vi "Debugl Loop Dialog.vi"(1 "Debug W1":u16, 2 "Debug W2":u16, 11 "error in (no error)":errorcluster) -> ()   [LabVIEW 2011]
uses:
  emi Lib/System 01/0 - General/App/Loop control/Private/_emi Loop status.ctl
  PCP interface/PCP Command Return.ctl
  PCP interface/PCP Commands.ctl
  emi Lib/System 01/0 - General/S&E reporting/Private/_emi_ S&E Message.ctl
  emi Lib/System 01/0 - General/S&E reporting/Private/_emi_ S&E Message type.ctl
  emi cndiates/E&S/Monitor/Actino S&E monitor.ctl
  PCP interface/PCP return data types/RDd return.ctl
  PCP interface/PCP return data types/RA return Analog I.ctl
  PCP interface/PCP return data types/RP return digital IO.ctl
  LEINmaster/Defenitions/LEIN CMD List.ctl
  Loop ID.ctl
  Measurments Handling/Action Analog Handler.ctl
  emi cndiates/E&S/String outpyt type.ctl
  PCP interface/PCP Command definer.ctl
  LEINmaster/Defenitions/LEIN Structure variations.ctl
  Options/Action GFV Settings.ctl
  Options/Options PageID.ctl
  emi Lib/System 01/0 - General/App/Loop control 2/Private/_emi_SMLoop Get State Single.vi
  emi Lib/System 01/0 - General/App/Loop control 2/Private/_emi_SMLoop Control Single.vi
  emi Lib/System 01/0 - General/App/Loop control 2/Private/_emi_ SMLoop start condition.vi
  emi Lib/System 01/0 - General/App/Loop control 2/Private/_emi_ SMLoop Error Check.vi
  emi Lib/Basic/0 - General/Error/emi_Is Error.vi
  emi Lib/System 01/0 - General/App/Loop control 2/Private/_emi_SMLoop Register new.vi
  emi Lib/Basic/0 - General/Data Types/emi_Enum Info.vi
  emi Lib/System 01/0 - General/S&E reporting/emi_Send S&E Error message.vi
  emi Lib/Basic/0 - General/Error/emi_ Is Error state.vi
  emi Lib/System 01/0 - General/emi_Read System ID.vi
  emi Lib/System 01/0 - General/App/Loop control/Private/_emi_GFV Loop Running.vi
  emi Lib/System 01/0 - General/App/Loop control/Private/_emi_GFV Loop Enable.vi
  emi Lib/System 01/0 - General/App/Loop control/Private/_emi_GFV Loop Linking.vi
  emi Lib/System 01/0 - General/App/Loop control 2/Private/_emi_ SMLoop Restart.vi
  emi Lib/System 01/0 - General/App/Loop control/Private/_emi_GFV stop a loop so it can reset.vi
  emi Lib/System 01/0 - General/App/Loop control 2/Private/_emi_ SMLoop Restart Counter.vi
  emi Lib/System 01/0 - General/App/Private/_emi_GFV App Close.vi
  emi Lib/System 01/0 - General/Private/_emi_GFV System ID.vi
  emi Lib/System 01/0 - General/S&E reporting/Private/_emi_S&E Q Generator.vi
  emi Lib/System 01/0 - General/Debug/Private/_emi_GFV Debug Disp.vi
  <vilib>/Utility/VariantDataType/GetNumericInfo.vi
  emi Lib/Basic/0 - General/Time/Private/emi_Time offset holder.vi
  emi Lib/System 01/0 - General/Debug/Private/_emi_GFV Debug Aditional.vi
  emi Lib/System 01/0 - General/Debug/Private/_emi_GFV Debug Log.vi
panel:
  in  "Tab Control":T1(tab)
  in  "Send to PCP":bool
  in  "d":dbl
  in  "n":i32
  out "PCP Ans Q. Element":i32
  out "PCP CMD Q. Element":i32
  out "latest notification":T2
  in  "Action":T3
  out "PCP Data out":T4
  out "ms since last data":u32
  in  "Empty":bool
  out "received/timedout 2":timestamp
  out "Valid reply":bool
  in  "Retry on err":bool=TRUE
  out "Receive ACK":bool
  out "motor timeout":bool
  out "Received command":T7
  out "motor returned":bool
  out "received/timedout":timestamp
  out "Received":u8[](array[numeric]) format="%02x"
  out "Time Stamp":timestamp
  out "Sent":u8[](array[numeric]) format="%02x"
  in  "To send (post A/S/T ID)":u8[](array[numeric]) format="%02x"
  in  "ACTI/STAT/TASK ID":u8 format="%02x"
  in  "CMD":T7
  in  "Sub node address":u8 format="%.0x"
  in  "Main controll address":u8=42
  in  "Send to sub node":bool
  in  "Send custom message":bool
  out "Til Tool cmd Q":i32
  out "Tool reply Q":i32
  in  "Sub Timeout (ms)":u16=200
  in  "priority":bool=TRUE
  out "S&E":T8[](array[typedef])
  in  "Action(GET)":T10=enum."Get All"
  in  "Type":T9
  out "size(s)":i32
  out "Alarma":string[](array[string])
  out "Errors":string[](array[string])
  in  "Test error Loop 2":errorcluster
  in  "Trigger 1":bool
  in  "Test error Loop 1":errorcluster
  out "error out":errorcluster
  out "Loops":T11[](array[typedef])
  # "Main controller Stroker: 42\nSolenoid: 16 \nPressure 1: 48 \nPressure 2: 49"
  # "X"
  # "X+1"
  # "X+2"
  # "X+3"
  # "X+4"
  # "X+5"
  # "X+6"
  # "X+7"
  # "X"
  # "X+1"
  # "X+2"
  # "X+3"
  # "X+4"
  # "X+5"
  # "X+6"
  # "X+7"
  # "X+8"
  # "X+9"
  # "X"
  # "X+1"
  # "X+2"
  # "X+3"
  # "X+4"
  # "X+5"
  # "X+6"
  # "X+7"
  # "X+8"
  # "X+9"
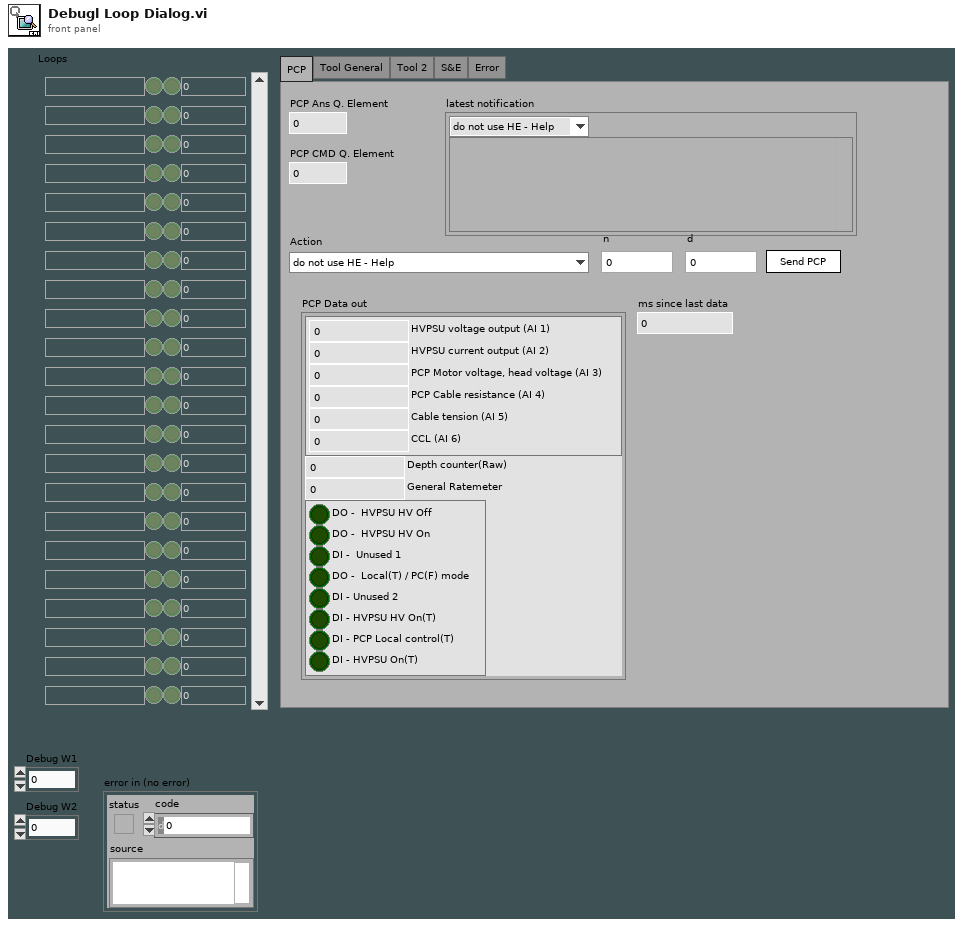
[diagram p1: front panel]
types:
  T1 = enum32{"PCP", "Tool General", "Tool 2", "S&E", "Error"}
  T2 = typedef "PCP Command Return.ctl" = cluster{"Action":T3, "Data in return":variant}
  T3 = typedef "PCP Commands.ctl" = enum16{"do not use HE - Help", "RDd - Most used inputs", "RA - All analog inputs", "RE n Reset DO n", "SE n Set DO n", "RP - Get digital inputs", "VA d Set AO A  Motor Volt", "VB d Set AO B  Cable Resistance", "VEr - Get Version", "DYp - Depth counter", "DR - Reset Depth Counter", "DS n Set Depth options(0-3)", "do not use ME - Manual mode enabled", "MD - Manual mode disabled", "ID - Get ID(2001)", "TS - Get Timestamp", "TO d(s)  Set timeout", "do not use LO n Start Loop Mode(1,2)", "AL n RD&LO variation", "ST - Stop Loop Mode"}
  T4 = typedef "RDd return.ctl" = cluster{"AI":T5, "Depth counter(Raw)":i32, "General Ratemeter":dbl, "Digital ports":T6}
  T5 = typedef "RA return Analog I.ctl" = cluster{"HVPSU voltage output (AI 1)":dbl, "HVPSU current output (AI 2)":dbl, "PCP Motor voltage, head voltage (AI 3)":dbl, "PCP Cable resistance (AI 4)":dbl, "Cable tension (AI 5)":dbl, "CCL (AI 6)":dbl}
  T6 = typedef "RP return digital IO.ctl" = cluster{"DO -  HVPSU HV Off":bool, "DO -  HVPSU HV On":bool, "DI -  Unused 1":bool, "DO -  Local(T) / PC(F) mode":bool, "DI - Unused 2":bool, "DI - HVPSU HV On(T)":bool, "DI - PCP Local control(T)":bool, "DI - HVPSU On(T)":bool}
  T7 = typedef "LEIN CMD List.ctl" = enum8{"ACTI", "TASK", "RES0", "STAT", "RES1", "RES2", "RES3", "USER"}
  T8 = typedef "_emi_ S&E Message.ctl" = cluster{"Type":T9, "Originate time":dbl, "System":u8, "Loop":u16, "Sub ID":u16, "Elevated priority":bool, "E&S Message content":variant}
  T9 = typedef "_emi_ S&E Message type.ctl" = enum16{"Error/Warning", "Note", "Debug", "Event", "Alarm Analog", "Alarm Digital", "Annotation"}
  T10 = typedef "Actino S&E monitor.ctl" = enum16{"GET(type history)", "SET S&E", "(Re)Init", "Get Error state", "Get  Alarm state", "Get All", "Get last  250", "Get Alarm History"}
  T11 = typedef "_emi Loop status.ctl" = cluster{"Loop Name":string, "Enabled":bool, "Running":bool, "Restarts":i32}
  T12 = typedef "Loop ID.ctl" = enum16{"Main-QSM", "Main-Dialog", "Main-Ind Upd", "Main-Graph Upd", "Main-Debug", "Main-DebugW1", "Main-DebugW2", "Main-SE Handler", "Interface-PCP", "Interface-CANbus", "Interface-Modem", "Var Handling-Beat", "Var Handling-From PCP", "Var Handling-File storage", "Var Handling-From Simulator", "GUI-GrphW Mast", "GUI-GrphW Slav", "SIM-Tool W1", "SIM-Tool W2", "Alm-Sound", "LEIN-motor", "Tool data gatherer Qer", "Tool Data LEIN STAT2 dekoder", "Indicator Value Update", "Tool STAT2 dedicated reader", "Tool ID handler", "Detail View L1", "Detail View L2", "Main display enable view", "Sequence runner", "Voltage setpoint", "Resistance setpoint", "Stroker Wizard L1", "Stroker Wizard L2", "Alarm Handling", "Annotations Tip Strip", "Magna Interface", "Modem Status", "Var Handling - Modem Status", "Power interface detector"}
  T13 = typedef "Action Analog Handler.ctl" = enum16{"GET value", "GET Single Frequenzy", "GET All Values", "GET Waveform", "Get Numb Var", "SET Value", "START Buffer", "REG Variable", "BUF size(total antal sekund)", "PULS", "Get a Value at time", "Set initial waveform"}
  T14 = typedef "String outpyt type.ctl" = enum16{"Full File hist", "Simple File hist", "Displ Hist one type", "Displ Hist mult types", "Displ Stat one type", "Displ Stat Mult type"}
  T15 = typedef "PCP Command definer.ctl" = cluster{"Action":T3, "n(0)":i32, "d(0.0)":dbl}
  T16 = typedef "LEIN Structure variations.ctl" = enum16{"LEIN08", "LEIN31", "LEIN63"}
  T17 = typedef "Action GFV Settings.ctl" = enum16{"Init", "Get From INI", "Put In INI", "Get Settings", "Get Update Index", "Set Setting"}
  T18 = typedef "Options PageID.ctl" = enum16{"P 1 (App)", "P 2", "P 3", "P 4", "P 5", "P 6 (Err)", "P 7 (Expert)", "P 8", "C 1", "C 2"}
  T19 = typedef "_emi_ SMLoop sates.ctl" = enum16{"Init", "Standby", "Start", "Normal Operation", "Stop", "Error Handling", "End", "Post"}
  T20 = typedef "LEIN CMD Cluster.ctl" = cluster{"SID":u8, "ANF":bool, "CMD":T7, "DATA":u8[]}
  T21 = typedef "LEIN custom reply Q.ctl" = refnum<queue>
  T22 = typedef "LEIN Reply Holder.ctl" = cluster{"Reply msg(cmdif no reply)":T20, "Reply time":timestamp, "Valid reply":bool}
  T23 = typedef "Options  All pages and custom.ctl" = cluster{"P 1 (App)":T24, "P 2":T25, "P 3":T26, "P 4":T29, "P 5":T34, "P 6 (Err)":T35, "P 7 (Expert)":T36, "P 8 (Depth)":T38, "C 1":T39, "C 2":T40}
  T24 = typedef "Options Page 1 (App).ctl" = cluster{"Result files":path, "PCP Interface":string, "Tractor/Stroker Interface":string, "Tractor Interface":string, "Modem Status Interface":string, "Audible Alarm":bool, "Force alarm on Technical":bool, "Force alarm on HH":bool, "Force alarm on LL":bool, "Force alarm on H":bool, "Force alarm on L":bool}
  T25 = typedef "Options Page 2.ctl" = cluster{"Solenoid & Relay latching time":u16, "Tractor relay 1":dbl, "Tractor relay 2":dbl, "Tractor Solenoid limit":dbl}
  T26 = typedef "Options Page 3.ctl" = cluster{"Min resistance":dbl, "Max resistance":dbl, "Head voltage range":T27, "Max voltage jump":dbl, "Maximum resistance change":dbl, "Start Telemetry Voltage":dbl, "Start Telemetry Timeout":dbl, "Start Motor Voltage":dbl, "Stop Motor Voltage":dbl, "Pass Mode Warning Voltage":dbl, "Relay Switch Voltage":dbl, "Relay Status Loss Voltage":dbl, "Samples to average":i32, "PSU type DO NOT USE":T28, "Magna OVP":dbl, "Magna Current Limit":dbl}
  T27 = typedef "PCP type List.ctl" = enum16{"0 - 350V", "0 - 450V", "0 - 600V"}
  T28 = typedef "PSU Type.ctl" = enum16{"Unipower", "Magna 8.3A", "Magna 12A", "None"}
  T29 = typedef "Options Page 4.ctl" = cluster{"Solenoid & Relay latching time":u16, "Stroker relay 1":dbl, "Stroker Relay 2":dbl, "Stroker Solenoid limit":dbl, "Force det.":T30, "Stroke force lim.":dbl, "Anchor Enabled Pressure":dbl, "Tacometer puls":dbl, "Default anchor behavior":T31, "Default stroker behavior":T32, "Default stroker force limit (tonne)":dbl, "Slips Size":T33}
  T30 = typedef "Stroke force selector.ctl" = enum16{"Stroke in = node 1", "Strok out = node 1"}
  T31 = typedef "Default anchor behavior.ctl" = enum16{"Do nothing", "Set Anchor", "Release Anchor"}
  T32 = typedef "Default stroker behavior.ctl" = enum16{"Do nothing", "Stop", "Go Out", "Go In"}
  T33 = typedef "Slips Type Radio.ctl" = enum32{"No Selection", "338 MRS", "3,9 MRS"}
  T34 = typedef "Options Page 5.ctl" = cluster{"Solenoid & Relay latching time":u16, "Driller relay 1":dbl, "Driller Relay 2":dbl, "Driller  Solenoid limit":dbl}
  T35 = typedef "Options Page 6 (Err).ctl" = cluster{"Error and event files":path}
  T36 = typedef "Options Page 7 (Expert).ctl" = cluster{"Show Debug":bool, "Log debug messages":bool, "Additional debug messages":bool, "Start Beagle with Simulator data":bool, "Workshop mode":bool, "Modem baud":u16, "enumCANCOM":bool, "Modem sim":T37, "Telemetry Timeout Disable":i32, "Buffer size":i32, "Upd regular data":bool, "Cable comp":cluster{"VMOD1 Voltage(V)":dbl, "VMOD2 Voltage(V)":dbl}}
  T37 = typedef "Modem simulation setup.ctl" = cluster{"Modem dealay sim":bool, "Sim baud Tx":u16, "Bit Error fraction Tx":dbl, "Sim baud Rx":u16, "Bit Error fraction Rx":dbl}
  T38 = typedef "Options Page 8 (Depth).ctl" = cluster{"Winch Spool Circumference":dbl, "Winch Pulses per Revolution":dbl, "Current Depth":dbl}
  T39 = typedef "Options Custom 1.ctl" = cluster{"Depth Updated":bool, "Depth Offset":dbl}
  T40 = typedef "Options Custom 2.ctl" = cluster{"Placeholder":bool}
  T41 = typedef "LVRectTypeDef.ctl" = cluster{"left":i16, "top":i16, "right":i16, "bottom":i16}
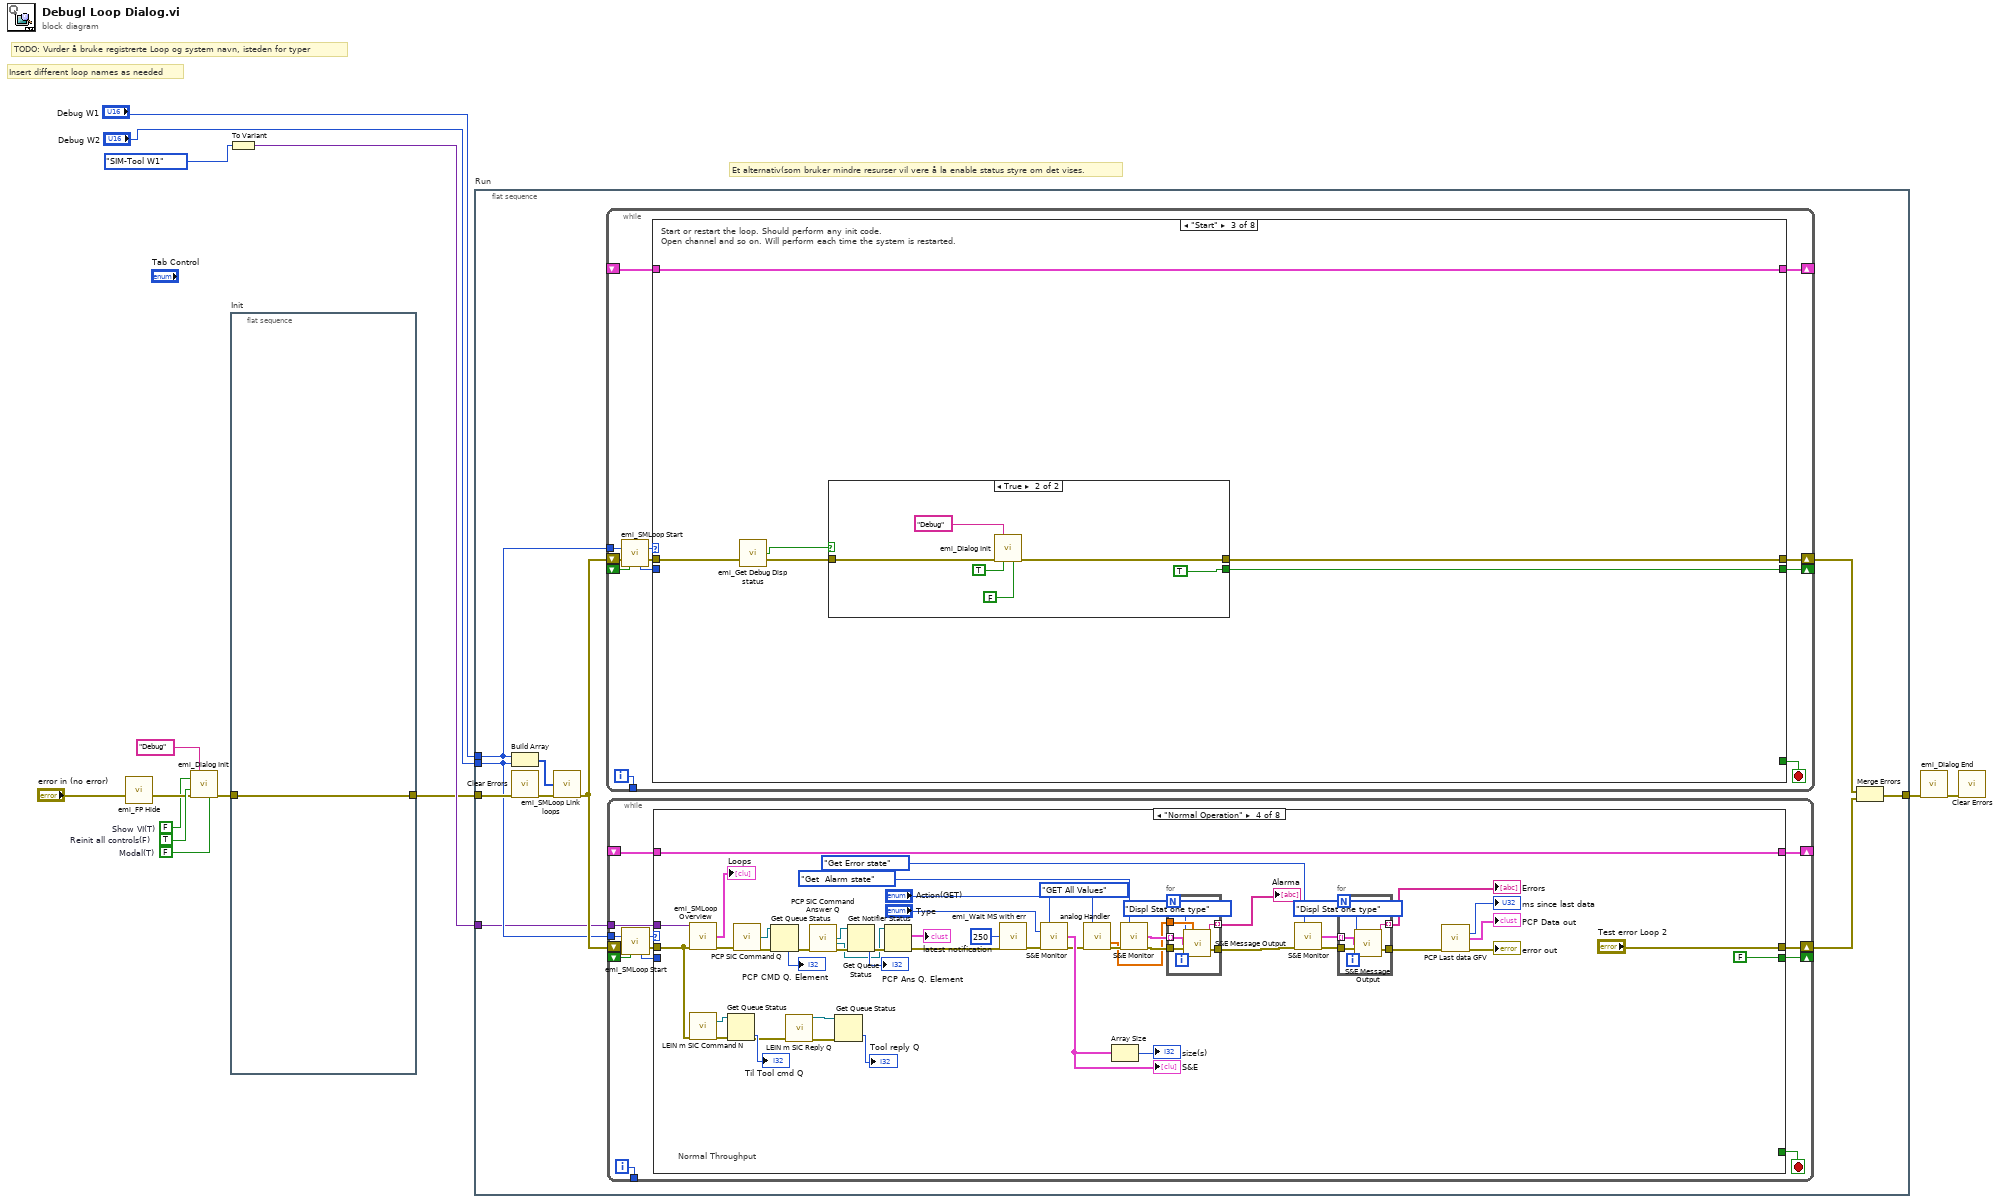
[diagram p0: block diagram]
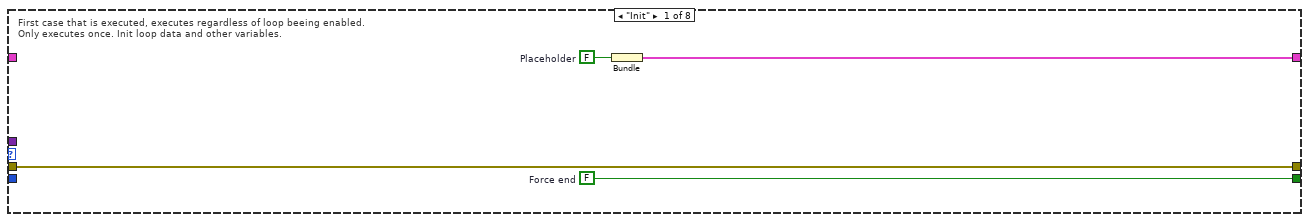
[diagram p2: hidden frame]
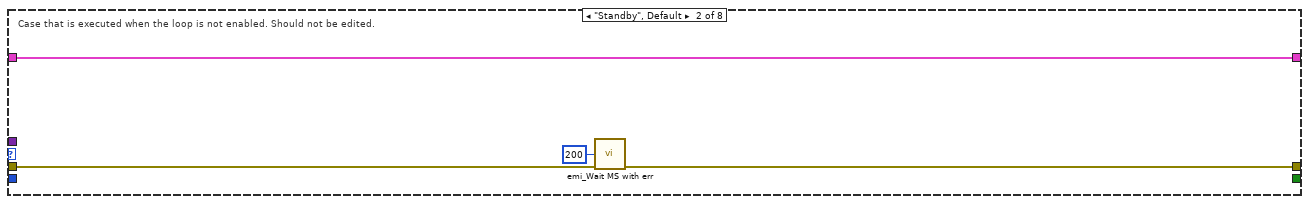
[diagram p3: hidden frame]
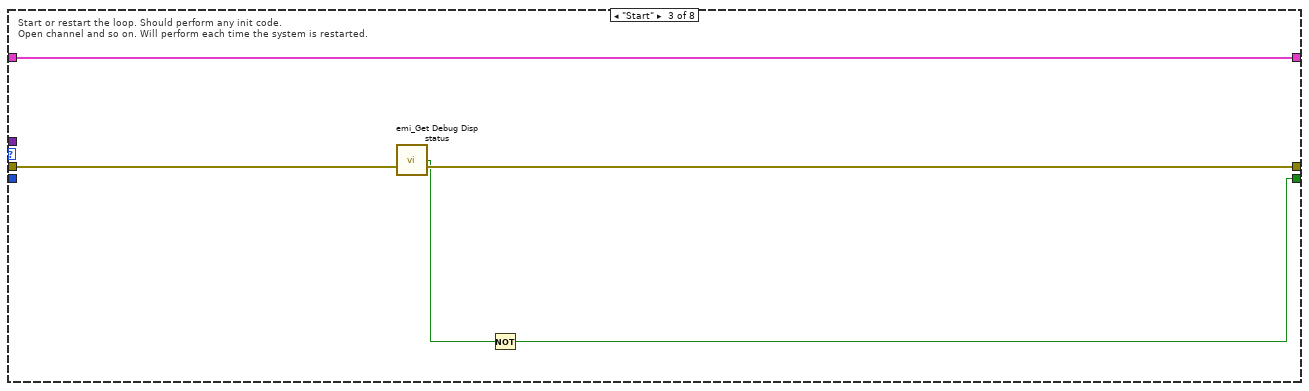
[diagram p4: hidden frame]
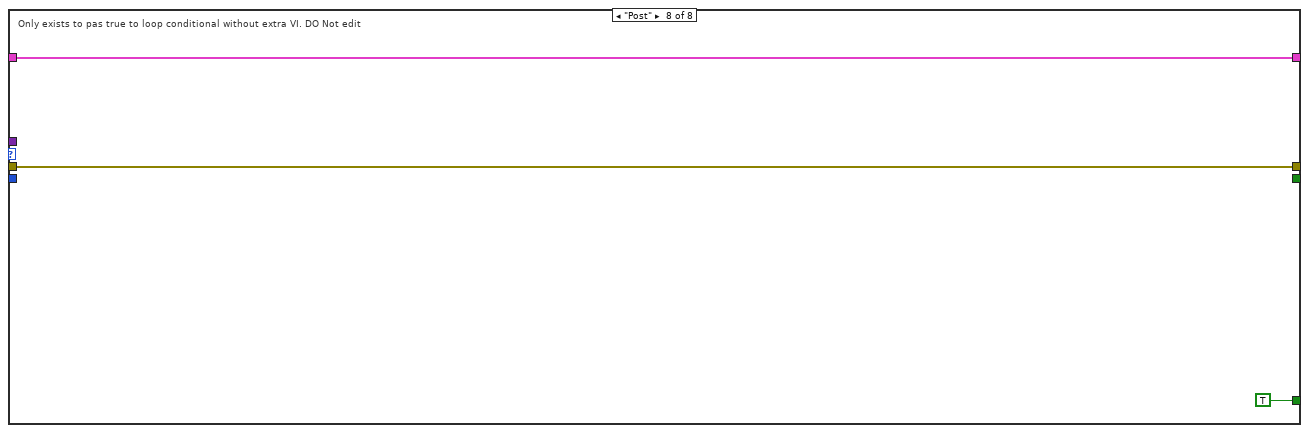
[diagram p8: hidden frame]
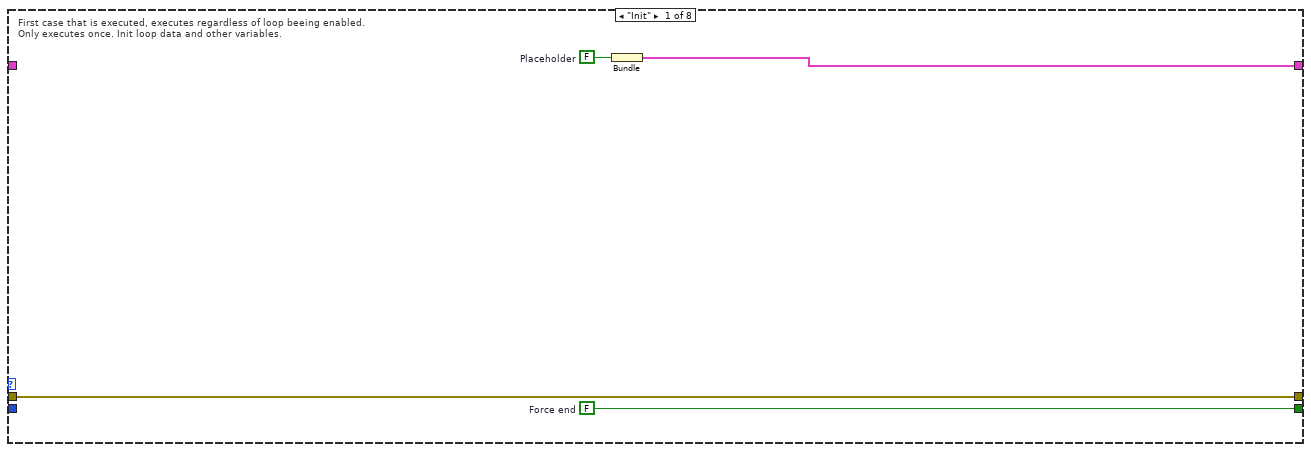
[diagram p9: hidden frame]
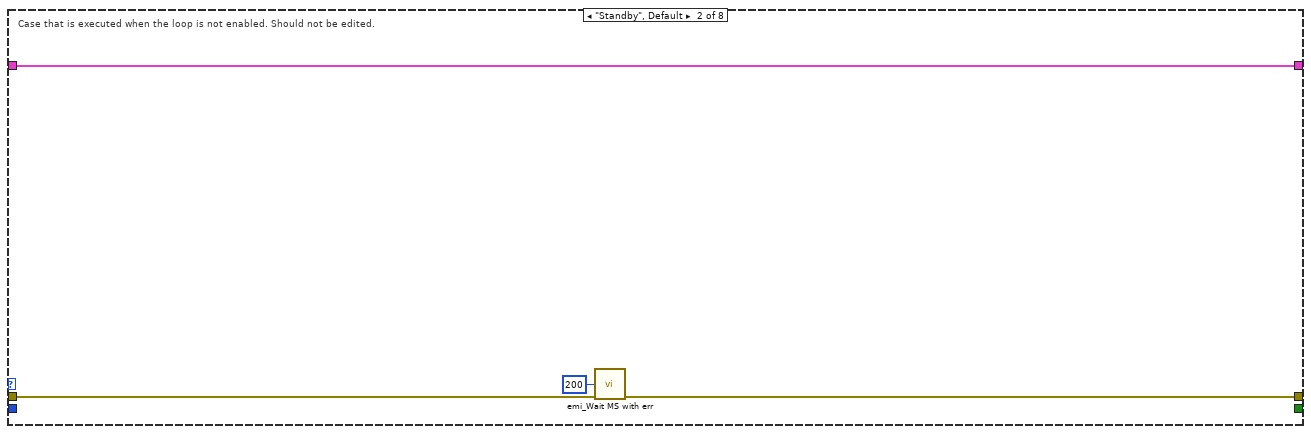
[diagram p10: hidden frame]
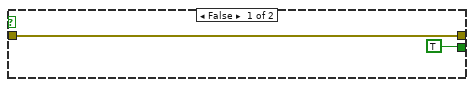
[diagram p11: hidden frame]
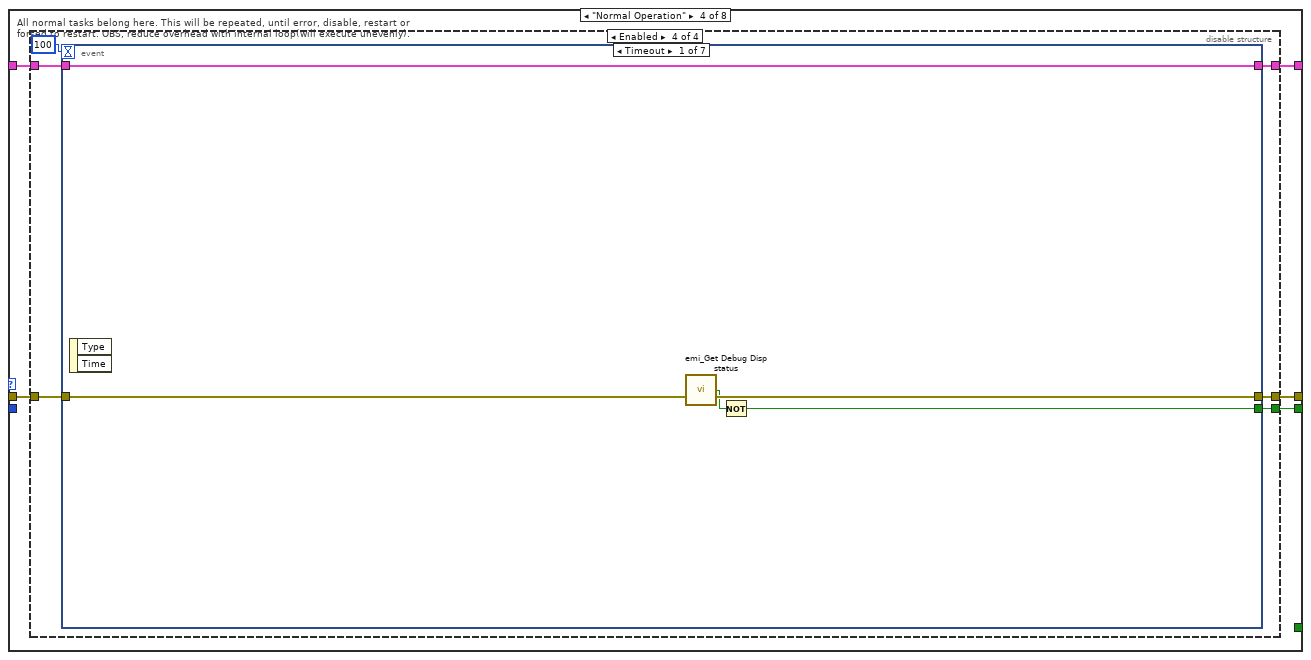
[diagram p12: hidden frame]
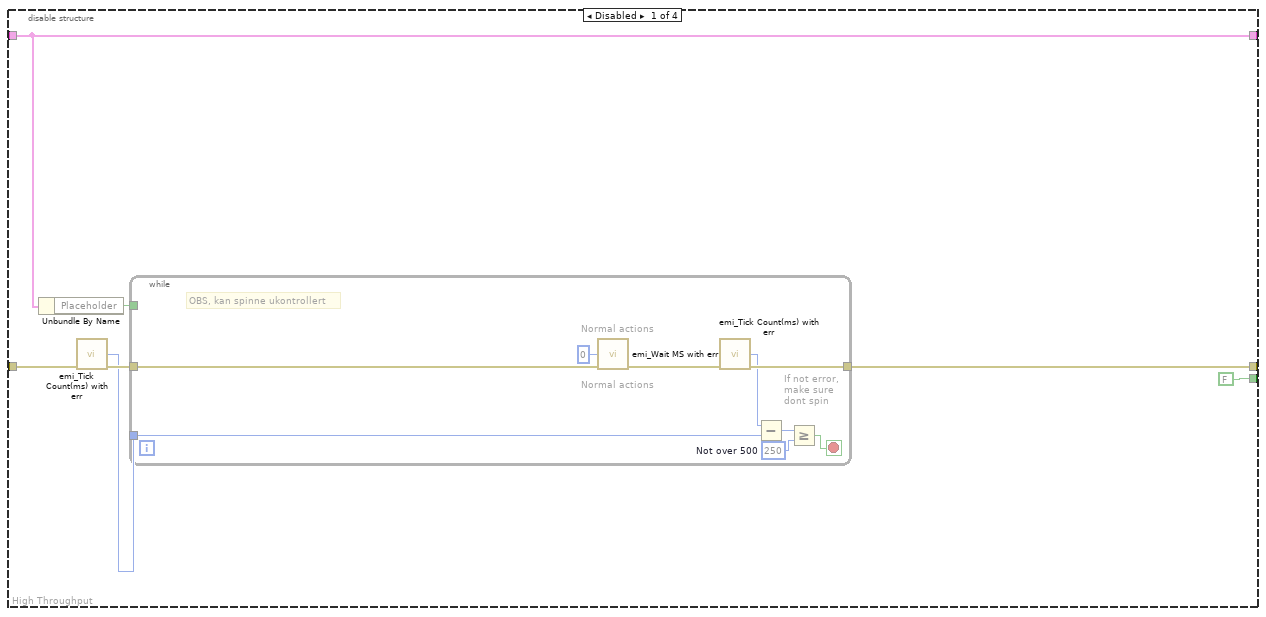
[diagram p13: hidden frame]
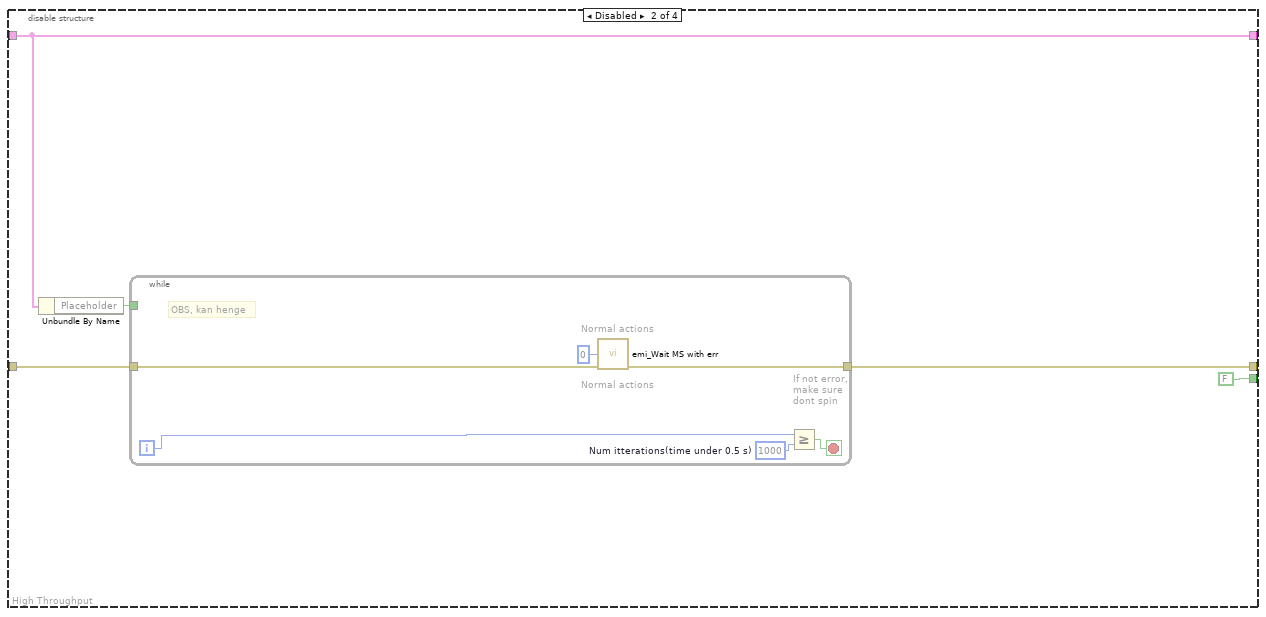
[diagram p14: hidden frame]
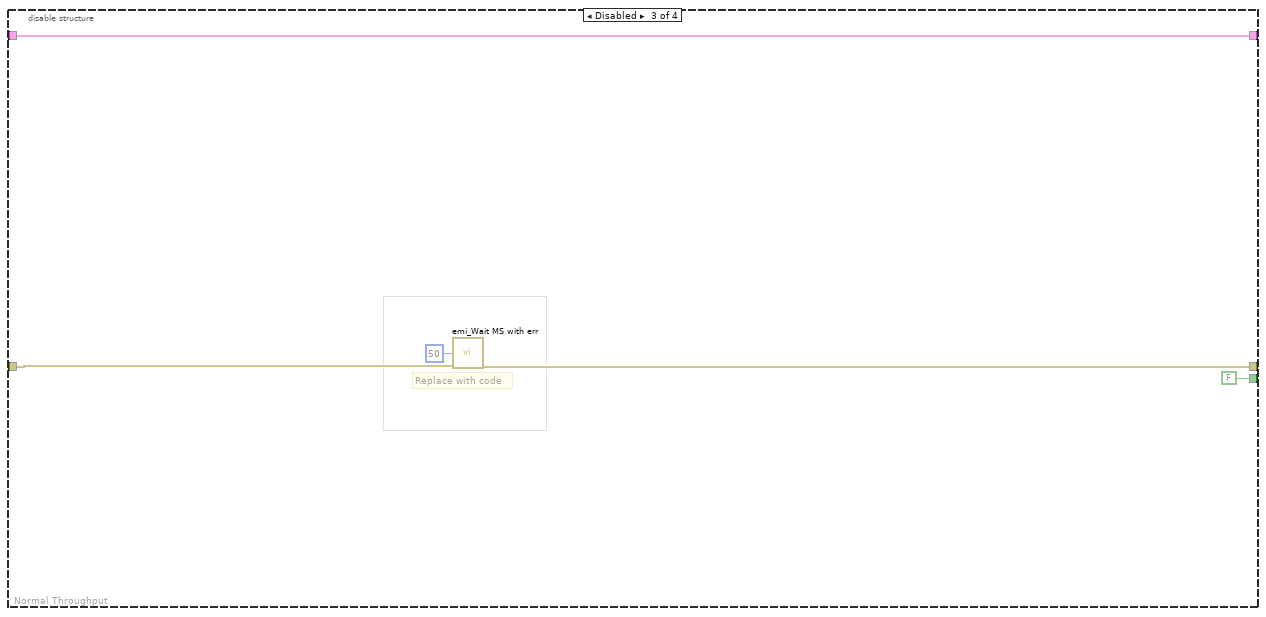
[diagram p15: hidden frame]
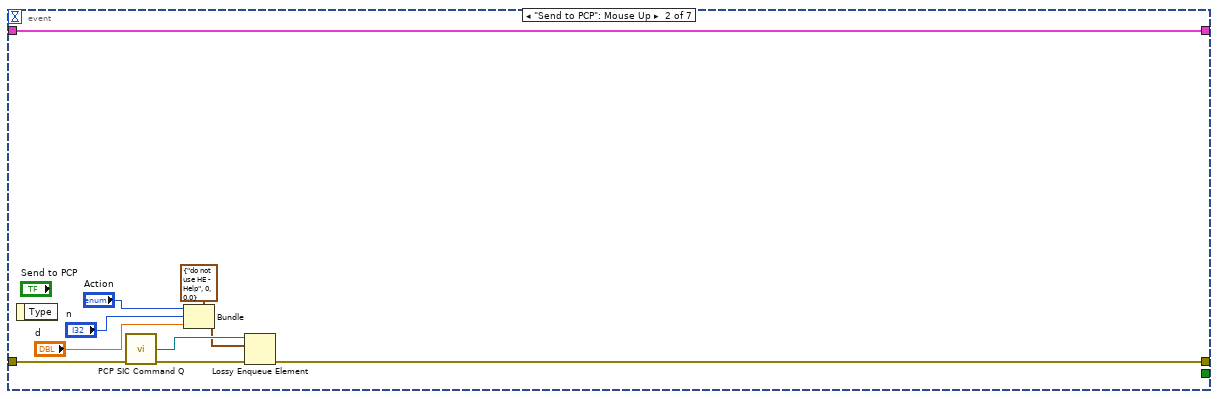
[diagram p16: hidden frame]
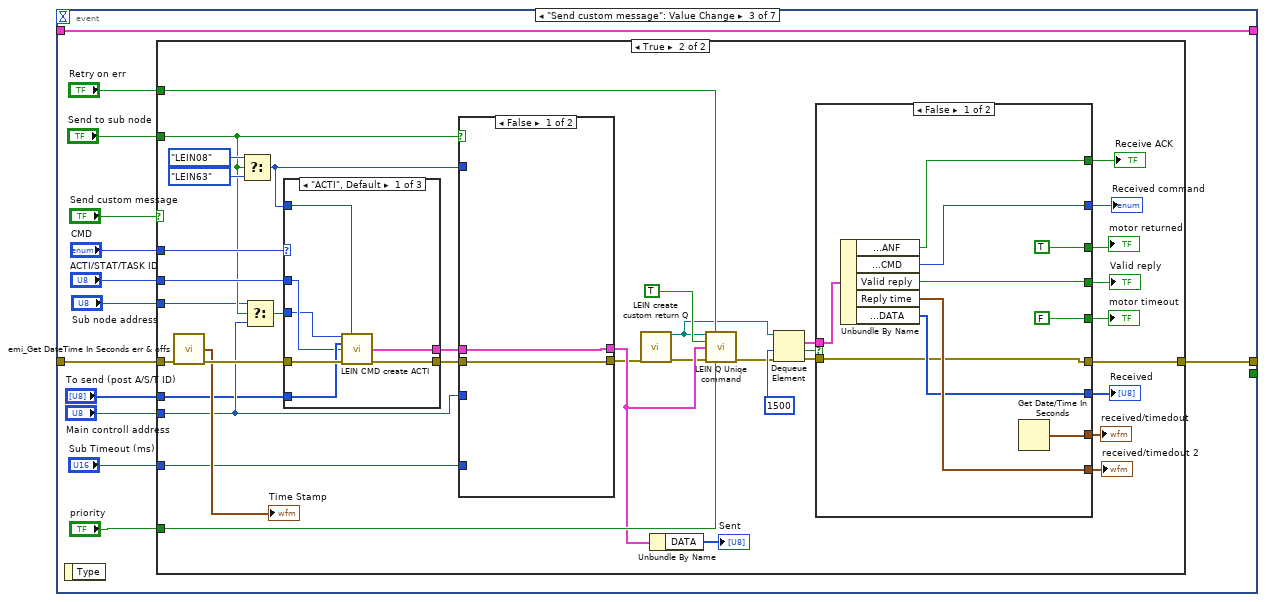
[diagram p17: hidden frame]
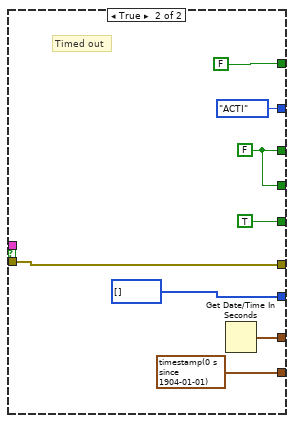
[diagram p19: hidden frame]
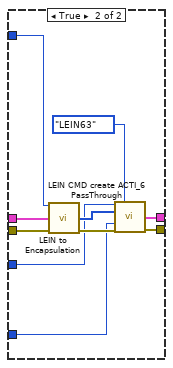
[diagram p20: hidden frame]
diagram:
  w9 = FALSE  # Show VI(T)
  w12 = TRUE  # Reinit all controls(F)
  w13 = FALSE  # Modal(T)
  # "Et alternativ(som bruker mindre resurser vil vere å la enable status styre om det vises."
  # "TODO: Vurder å bruke registrerte Loop og system navn, isteden for typer"
  # "Insert different loop names as needed"
  n1 = call "emi_FP Hide.vi"("error in (no error)"="error in (no error)") -> ("error out"=w11:errorcluster)  [unwired: 13 in, 1 out]
  n2 = call "emi_Dialog Init.vi"("Header String(\"\")"="Debug" ("Header String(\"\")"), "Show VI(T)"=w9, "Reinit all controls(F)"=w12, "error in"=w11, "Modal(T)"=w13) -> ("error out"=w10:errorcluster)  [unwired: 10 in]
  n3 = To Variant(anything=Loop_ID."SIM-Tool W1" ("Loop ID")) -> (Variant=w7:variant)
  n4 = flat-sequence "Init" {
    tunnel: [w15] -> w5
    tunnel: w10 -> [w15]
    frame #0 {
    }
  }
  n5 = flat-sequence "Run" {
    tunnel: w5 -> [w25]
    tunnel: [w22] -> w8
    tunnel: "Debug W1" -> [w19]
    tunnel: "Debug W2" -> [w18]
    tunnel: w7 -> [w16]
    frame #0 {
      n6 = Build Array(w19, w18) -> (w17:u16[])
      n7 = call <vilib>:"Clear Errors.vi"("error in (no error)"=w25) -> ("error out"=w21:errorcluster)  [unwired: 6 in]
      n8 = call "emi_SMLoop Link loops.vi"("Loop IDS"=w17, "error in (no error)"=w21) -> ("error out"=w20:errorcluster)  [unwired: 13 in]
      n9 = while {
        shift-right: [w131] -> _
        shift-left: _ -> [w127]
        shift-right: [w129] -> w24
        shift-left: w20 -> [w125]
        tunnel: [w128] -> _
        shift-right: [w126] -> _
        shift-left: _ -> [w121]
        tunnel: w19 -> [w122]
        i -> [w128]
        stop <- w130 stop-if-true
        n10 = call "emi_SMLoop Start.vi"("Loop ID"=w122, "error in (no error)"=w125, "Force Stop(F)"=w121) -> ("Loop command"=w123:T19, "error out"=w124:errorcluster, "Loop ID out"=w120:i32)  [unwired: 10 in]
        n11 = case shown="\"Start\"" w123 {
          tunnel: [w134 w136 w145 w156 w385 w392 w393 w396] -> w131
          tunnel: [_ _ _ _ _ _ _ TRUE] -> w130
          tunnel: w124 -> [w135 w138 w143 w158 w384 w391 w394 w397]
          tunnel: [w135 w137 w144 w157 w375 w391 w394 w397] -> w129
          tunnel: w127 -> [_ w136 w145 w155 w385 w392 w393 w396]
          tunnel: [w132 _ w140 w154 _ _ _ _] -> w126
          tunnel: w120 -> [_ _ _ _ w383 _ _ _]
          frame "Init" {
            w132 = FALSE  # Force end
            w133 = FALSE  # Placeholder
            # "First case that is executed, executes regardless of loop beeing enabled.\nOnly executes once. Init loop data and other variables."
            n12 = Bundle("Placeholder"=w133) -> (w134:cluster{"Placeholder":bool})  [unwired: 1 in]
          }
          frame "Standby", Default {
            # "Case that is executed when the loop is not enabled. Should not be edited."
            n13 = call "emi_Wait MS with err.vi"("milliseconds to wait(0)"=u32 200, "error in (no error)"=w138) -> ("error out"=w137:errorcluster)  [unwired: 13 in]
          }
          frame "Start" {
            # "Start or restart the loop. Should perform any init code. \nOpen channel and so on. Will perform each time the system is restarted."
            n14 = call "emi_Get Debug Disp status.vi"("error in (no error)"=w143) -> ("Debug Disp"=w141:bool, "error out"=w142:errorcluster)  [unwired: 13 in]
            n15 = case shown="True" w141 {
              tunnel: [w147 w153] -> w144
              tunnel: w142 -> [w147 w152]
              tunnel: [TRUE ("Discard?") TRUE ("Discard?")] -> w140
              frame False {
              }
              frame True {
                n16 = call "emi_Dialog Init.vi"("Header String(\"\")"="Debug" ("Header String(\"\")"), "error in"=w152, "Center in bottom FP(T)"=TRUE, "Modal(T)"=FALSE ("Set BG Color(T)")) -> ("error out"=w153:errorcluster)  [unwired: 11 in]
              }
            }
          }
          frame "Normal Operation" {
            # "All normal tasks belong here. This will be repeated, until error, disable, restart or\nforsed to restart. OBS, reduce overhead with internal loop(will execute unevenly)."
            n17 = disable-structure shown="Enabled" {
              disable-tunnel: w158 -> [w162 w175 w188 w196]
              disable-tunnel: [w164 w178 w187 w192] -> w157
              disable-tunnel: [w165 w179 w190 w193] -> w156
              disable-tunnel: w155 -> [w165 w179 w190 w194]
              disable-tunnel: [FALSE ("Force End") FALSE ("Force End") FALSE ("Force End") w191] -> w154
              frame Disabled {
                # "High Throughput"
                n18 = Unbundle By Name(w165) -> ("Placeholder"=w163:bool)
                n19 = call "emi_Tick Count(ms) with err.vi"("error in (no error)"=w162) -> ("millisecond timer value"=w160:u32, "error out"=w161:errorcluster)  [unwired: 13 in]
                n20 = while {
                  tunnel: w161 -> [w168]
                  tunnel: [w174] -> w164
                  tunnel: w163 -> [_]
                  tunnel: w160 -> [w173]
                  stop <- w167 stop-if-true
                  w170 = u32 250  # Not over 500
                  # "OBS, kan spinne ukontrollert"
                  # "If not error,\nmake sure \ndont spin"
                  # "Normal actions"
                  # "Normal actions"
                  n21 = call "emi_Wait MS with err.vi"("milliseconds to wait(0)"=u32 0, "error in (no error)"=w168) -> ("error out"=w169:errorcluster)  [unwired: 13 in]
                  n22 = call "emi_Tick Count(ms) with err.vi"("error in (no error)"=w169) -> ("millisecond timer value"=w172:u32, "error out"=w174:errorcluster)  [unwired: 13 in]
                  n23 = Subtract(x=w172, y=w173) -> (x-y=w171:u32)
                  n24 = Greater Or Equal?(x=w171, y=w170) -> (x >= y?=w167:bool)
                }
              }
              frame Disabled {
                # "High Throughput"
                n25 = Unbundle By Name(w179) -> ("Placeholder"=w177:bool)
                n26 = while {
                  tunnel: [w181] -> w178
                  tunnel: w177 -> [_]
                  tunnel: w175 -> [w182]
                  i -> [w180]
                  stop <- w184 stop-if-true
                  w185 = u32 1000  # Num itterations(time under 0.5 s)
                  # "OBS, kan henge"
                  # "If not error,\nmake sure \ndont spin"
                  # "Normal actions"
                  # "Normal actions"
                  n27 = call "emi_Wait MS with err.vi"("milliseconds to wait(0)"=u32 0, "error in (no error)"=w182) -> ("error out"=w181:errorcluster)  [unwired: 13 in]
                  n28 = Greater Or Equal?(x=w180, y=w185) -> (x >= y?=w184:bool)
                }
              }
              frame Disabled {
                # "Replace with code"
                # "Normal Throughput"
                n29 = call "emi_Wait MS with err.vi"("milliseconds to wait(0)"=u32 50, "error in (no error)"=w188) -> ("error out"=w187:errorcluster)  [unwired: 13 in]
              }
              frame Enabled {
                n30 = event shown="[0] Timeout" {
                  selector: _ -> [_ _ _ _ _ _ _]
                  dyn-events: _ -> [_ _ _ _ _ _ _]
                  timeout: 100 -> [_ _ _ _ _ _ _]
                  tunnel: w196 -> [w200 w210 w223 w326 w333 w360 w369]
                  tunnel: w194 -> [w201 w211 w224 w328 w334 w363 w371]
                  tunnel: [w201 w211 w224 w328 w334 w363 w371] -> w193
                  tunnel: [w199 w208 w221 w317 w331 w361 w370] -> w192
                  tunnel: [w197 _ _ w327 _ _ _] -> w191
                  event Timeout {
                    n31 = event-data() -> ()  [unwired: 1 in, 2 out]
                    n32 = call "emi_Get Debug Disp status.vi"("error in (no error)"=w200) -> ("Debug Disp"=w198:bool, "error out"=w199:errorcluster)  [unwired: 13 in]
                    n33 = Not(x=w198) -> (.not. x?=w197:bool)
                  }
                  event "Send to PCP": Mouse Up {
                    n34 = event-data() -> ()  [unwired: 1 in, 1 out]
                    n35 = call "PCP SIC Command Q.vi"("error in (no error)"=w210) -> ("PCP cmd Q"=w207:refnum<queue>, "error out"=w209:errorcluster)  [unwired: 13 in]
                    n36 = Bundle(cluster=T15 {"Action"=enum."do not use HE - Help", "n(0)"=0, "d(0.0)"=0.0} ("element"), "Action"="Action", "n(0)"="n", "d(0.0)"="d") -> (w205:T15)
                    n37 = Lossy Enqueue Element(queue=w207, element=w205, error in (no error)=w209) -> (error out=w208:errorcluster)  [unwired: 3 out]
                  }
                  event "Send custom message": Value Change {
                    n38 = event-data() -> ()  [unwired: 1 in, 1 out]
                    n39 = case shown="True" "Send custom message" {
                      tunnel: w223 -> [w225 w260]
                      tunnel: [w225 w236] -> w221
                      tunnel: "Send to sub node" -> [_ w253]
                      tunnel: "CMD" -> [_ w256]
                      tunnel: "ACTI/STAT/TASK ID" -> [_ w254]
                      tunnel: "Main controll address" -> [_ w252]
                      tunnel: "Sub node address" -> [_ w251]
                      tunnel: "To send (post A/S/T ID)" -> [_ w249]
                      tunnel: "Sub Timeout (ms)" -> [_ w248]
                      tunnel: "priority" -> [_ w246]
                      tunnel: "Retry on err" -> [_ w245]
                      frame False {
                      }
                      frame True {
                        n40 = call "emi_Get DateTime In Seconds err & offs.vi"("error in (no error)"=w260) -> ("Time"=→"Time Stamp":timestamp, "error out"=w259:errorcluster)  [unwired: 13 in]
                        n41 = Select(t=LEIN_Structure_variations."LEIN08" ("LEIN Variation"), s=w253, f=LEIN_Structure_variations."LEIN63" ("LEIN Variation")) -> (s? t:f=w255:T16)
                        n42 = Select(t=w251, s=w253, f=w252) -> (s? t:f=w250:u8)
                        n43 = case shown="\"ACTI\", Default" w256 {
                          tunnel: [w299 w307 w314] -> w263
                          tunnel: [w298 w306 w313] -> w262
                          tunnel: w259 -> [w300 w305 w315]
                          tunnel: w255 -> [w297 w304 _]
                          tunnel: w254 -> [w295 w303 w308]
                          tunnel: w250 -> [w294 w302 w312]
                          tunnel: w249 -> [w296 w301 _]
                          frame "ACTI", Default {
                            n44 = call "LEIN CMD create ACTI.vi"("SID"=w294, "LEIN Variation"=w297, "Data"=w296, "ACTI ID"=w295, "error in (no error)"=w300) -> ("CMD"=w298:T20, "error out"=w299:errorcluster)  [unwired: 9 in]
                          }
                          frame "TASK" {
                            n45 = call "LEIN CMD create Task.vi"("SID"=w302, "LEIN Variation"=w304, "Data"=w301, "TASK ID"=w303, "error in (no error)"=w305) -> ("CMD"=w306:T20, "error out"=w307:errorcluster)  [unwired: 9 in]
                          }
                          frame "STAT" {
                            n46 = Quotient & Remainder(x=w308, y=u8 16) -> (x-y*floor(x/y)=w309:u8, floor(x/y)=w310:u8)
                            n47 = call "LEIN CMD create STAT.vi"("SID"=w312, "STAT ID"=w310, "STAT Part"=w309, "error in (no error)"=w315) -> ("CMD"=w313:T20, "error out"=w314:errorcluster)  [unwired: 10 in]
                          }
                        }
                        n48 = case shown="False" w253 {
                          tunnel: [w282 w290] -> w243
                          tunnel: [w283 w289] -> w242
                          tunnel: w263 -> [w283 w288]
                          tunnel: w262 -> [w282 w287]
                          tunnel: w252 -> [_ w286]
                          tunnel: w255 -> [_ w285]
                          tunnel: w248 -> [_ w284]
                          frame False {
                          }
                          frame True {
                            n49 = call "LEIN to Encapsulation.vi"("LEIN Variation"=w285, "CMD"=w287, "error in (no error)"=w288) -> ("Data and header"=w291:u8[], "error out"=w292:errorcluster)  [unwired: 8 in, 3 out]
                            n50 = call "LEIN CMD create ACTI_6 PassThrough.vi"("SID"=w286, "LEIN Variation"=LEIN_Structure_variations."LEIN63", "LEIN ecapsulated data (header and data)"=w291, "Sub Timeout (ms)"=w284, "error in (no error)"=w292) -> ("CMD"=w290:T20, "error out"=w289:errorcluster)  [unwired: 9 in]
                          }
                        }
                        n51 = call "LEIN create custom return Q.vi"("error in (no error)"=w242) -> ("LEIN custom reply Q"=w238:T21, "error out"=w241:errorcluster)  [unwired: 13 in]
                        n52 = Unbundle By Name(w243) -> ("DATA"=→"Sent":u8[])
                        n53 = call "LEIN Q Uniqe command.vi"("LEIN custom reply Q"=w238, "Retry on err (F)"=w245, "Custom Q(F)"=TRUE, "CMD"=w243, "error in"=w241, "priority(F)"=w246) -> ("error out"=w239:errorcluster)  [unwired: 9 in]
                        n54 = Dequeue Element(queue=w238, timeout in ms (-1)=1500, error in (no error)=w239) -> (element=w230:T22, timed out?=w234:bool, error out=w237:errorcluster)  [unwired: 1 out]
                        n55 = case shown="False" w234 {
                          tunnel: w237 -> [w264 w281]
                          tunnel: [w264 w281] -> w236
                          tunnel: [w273 w280] -> w235
                          tunnel: [TRUE ("Received") w279] -> w233
                          tunnel: [w269 w279] -> w232
                          tunnel: [FALSE ("Received") TRUE ("Received")] -> w231
                          tunnel: w230 -> [w270 _]
                          tunnel: [w268 LEIN_CMD_List."ACTI" ("CMD")] -> w229
                          tunnel: [w267 timestamp(0 s since 1904-01-01) ("received/timedout 2")] -> w228
                          tunnel: [w266 FALSE ("ANF")] -> w227
                          tunnel: [w265 u8[] [] ("DATA")] -> w226
                          frame False {
                            n56 = Unbundle By Name(w270) -> ("Reply msg(cmdif no reply).ANF"=w266:bool, "Reply msg(cmdif no reply).CMD"=w268:T7, "Valid reply"=w269:bool, "Reply time"=w267:timestamp, "Reply msg(cmdif no reply).DATA"=w265:u8[])
                            n57 = Get Date/Time In Seconds() -> (seconds since 1Jan1904=w273:timestamp)
                          }
                          frame True {
                            w279 = FALSE ("Received")
                            # "Timed out"
                            n58 = Get Date/Time In Seconds() -> (seconds since 1Jan1904=w280:timestamp)
                          }
                        }
                        "received/timedout" <- w235
                        "Valid reply" <- w232
                        "motor timeout" <- w231
                        "motor returned" <- w233
                        "Received command" <- w229
                        "received/timedout 2" <- w228
                        "Receive ACK" <- w227
                        "Received" <- w226
                      }
                    }
                  }
                  event Panel Close? {
                    w327 = TRUE ("Discard?")
                    # "Ellers varierer det om \nDebug Synlig/ikke Synlig huskes(\nalt etter om options vises etterpå)"
                    n59 = event-data() -> ()  [unwired: 1 in, 3 out]
                    n60 = call "Options GFV.vi"("error in (no error)"=w326, "Action(Get Settings)"=Action_GFV_Settings."Get Settings") -> ("Options"=w321:T23, "error out"=w323:errorcluster)  [unwired: 15 in, 1 out]
                    n61 = Unbundle By Name(w321) -> ("P 7 (Expert)"=w320:T36)
                    n62 = in-place {
                      n63 = in-place-cluster #1(w320) -> ()  [unwired: 1 out]
                      n64 = in-place-cluster #1("Show Debug"=FALSE) -> (w319:T36)
                    }
                    n65 = call "Options GFV.vi"("Anything"=w319, "error in (no error)"=w323, "Action(Get Settings)"=Action_GFV_Settings."Set Setting", "Setting ID"=Options_PageID."P 7 (Expert)") -> ("error out"=w318:errorcluster)  [unwired: 13 in, 2 out]
                    n66 = call "Options GFV.vi"("error in (no error)"=w318, "Action(Get Settings)"=Action_GFV_Settings."Put In INI") -> ("error out"=w317:errorcluster)  [unwired: 15 in, 2 out]
                    n67 = event-data("Discard?"=w327) -> ()  [unwired: 1 in, 1 out]
                  }
                  event "Loops": Mouse Down {
                    n68 = event-data() -> ("Coords.Vertical"=w332:i32, "Mods.Double Click"=w330:bool)  [unwired: 1 in]
                    n69 = case shown="True" w330 {
                      tunnel: w333 -> [w335 w358]
                      tunnel: w332 -> [_ w351]
                      tunnel: [w335 w339] -> w331
                      frame False {
                      }
                      frame True {
                        n70 = control-ref of="Loops"() -> (w359:refnum<vi>)
                        n71 = property class="Arr (strict)"(reference=w359, error in=w358) -> (reference out=w355:refnum<vi>, error out=w356:errorcluster, "MasterRect"=w357:T41, "Number of Rows"=w352:u32, "Index Values"=w338:u32[])
                        n72 = Index Array(array=w338) -> (element=w336:u32)  [unwired: 1 in]
                        n73 = Close Reference(reference=w355, error in (no error)=w356) -> (error out=w345:errorcluster)
                        n74 = Unbundle By Name(w357) -> ("bottom"=w354:i16, "top"=w350:i16)
                        n75 = Subtract(x=w354, y=w350) -> (x-y=w353:i16)
                        n76 = Subtract(x=w351, y=w350) -> (x-y=w349:i32)
                        n77 = Divide(x=w353, y=w352) -> (x/y=w348:dbl)
                        n78 = Divide(x=w349, y=w348) -> (x/y=w346:dbl)
                        n79 = Round Toward -Infinity(1:w346) -> (0:w347:dbl)
                        n80 = To Long Integer(number=w347) -> (32bit integer=w344:i32)
                        n81 = Add(x=w344, y=w336) -> (x+y=w337:u32)
                        n82 = call-poly "emi_SMLoop Get State.vi"("Loop ID in"=w337, "error in (no error)"=w345) -> ("Loop ID out"=w343:u16, "error out"=w342:errorcluster, "Loop Enable Out"=w341:bool)  [unwired: 7 in, 4 out]
                        n83 = Not(x=w341) -> (.not. x?=w340:bool)
                        n84 = call-poly "emi_SMLoop Control.vi"("Loop ID in"=w343, "Enable"=w340, "error in (no error)"=w342) -> ("error out"=w339:errorcluster)  [unwired: 11 in, 1 out]
                      }
                    }
                  }
                  event "Trigger 1": Value Change {
                    n85 = event-data() -> ()  [unwired: 1 in, 1 out]
                    n86 = case shown="True" "Trigger 1" {
                      tunnel: [w364 w366] -> w361
                      tunnel: w360 -> [w364 w367]
                      frame False {
                      }
                      frame True {
                        n87 = Merge Errors(w367, "Test error Loop 1") -> (w366:errorcluster)
                      }
                    }
                  }
                  event "Empty": Value Change {
                    n88 = event-data() -> ("NewVal"=w368:bool)  [unwired: 1 in]
                    n89 = case shown="True" w368 {
                      tunnel: [w372 w374] -> w370
                      tunnel: w369 -> [w372 w374]
                      frame False {
                      }
                      frame True {
                        n90 = local write "To send (post A/S/T ID)"(i32[] [] ("To send (post A/S/T ID)")) -> ()
                      }
                    }
                  }
                }
              }
            }
          }
          frame "Stop" {
            # "Så ikke auto starter igjen om enablet"
            # "To alow VI to exit befor \nAplicatin End.\nFor use in dialogs"
            # "Stop the loop. May be restarted later. Close interfaces and the like"
            n91 = disable-structure shown="Enabled" {
              disable-tunnel: w384 -> [w389 w390]
              disable-tunnel: w383 -> [w388 _]
              disable-tunnel: [w386 w390] -> w382
              frame Enabled {
                n92 = call-poly "emi_SMLoop Control.vi"("Loop ID in"=w388, "Enable"=FALSE, "error in (no error)"=w389) -> ("error out"=w386:errorcluster)  [unwired: 11 in, 1 out]
              }
              frame Disabled {
              }
            }
            n93 = call "emi_FP Hide.vi"("error in (no error)"=w382) -> ("error out"=w376:errorcluster)  [unwired: 13 in, 1 out]
            n94 = call "emi_Get Debug Aditional status.vi"("error in (no error)"=w376) -> ("Debug Additional"=w378:bool, "error out"=w381:errorcluster)  [unwired: 13 in]
            n95 = call "emi_Get Debug Log status.vi"("error in (no error)"=w381) -> ("Debug Log"=w379:bool, "error out"=w380:errorcluster)  [unwired: 13 in]
            n96 = call "emi_Set Debug status.vi"("Debug Disp"=FALSE, "Debug Log"=w379, "Debug Aditional"=w378, "error in (no error)"=w380) -> ("error out"=w375:errorcluster)  [unwired: 11 in]
          }
          frame "Error Handling" {
            # "Loop automaticaly returns here after error is found. If error is cleared, \nLoop wil continue as normal(if was operative when error."
          }
          frame "End" {
            # "Only executes at application end has. Should performa any action the loop \nneeds to finnish. Executes only once."
          }
          frame "Post" {
            # "Only exists to pas true to loop conditional without extra VI. DO Not edit"
          }
        }
      }
      n97 = while {
        shift-right: [w38] -> _
        shift-left: _ -> [w34]
        shift-right: [w36] -> w23
        shift-left: w20 -> [w32]
        tunnel: [w35] -> _
        shift-right: [w33] -> _
        shift-left: _ -> [w28]
        tunnel: w18 -> [w29]
        tunnel: w16 -> [w26]
        i -> [w35]
        stop <- w37 stop-if-true
        n98 = call "emi_SMLoop Start.vi"("Loop ID"=w29, "error in (no error)"=w32, "Force Stop(F)"=w28) -> ("Loop command"=w30:T19, "error out"=w31:errorcluster, "Loop ID out"=w27:i32)  [unwired: 10 in]
        n99 = case shown="\"Normal Operation\"" w30 {
          tunnel: [w42 w43 w51 w97 w111 w114 w115 w118] -> w38
          tunnel: [_ _ _ _ _ _ _ TRUE] -> w37
          tunnel: w31 -> [w39 w45 w50 w99 w112 w113 w116 w119]
          tunnel: [w39 w44 w49 "Test error Loop 2" w112 w113 w116 w119] -> w36
          tunnel: w34 -> [_ w43 w51 w97 w111 w114 w115 w118]
          tunnel: [w40 _ w47 FALSE ("Force End") _ _ _ _] -> w33
          tunnel: w27 -> [_ _ _ _ _ _ _ _]
          tunnel: w26 -> [_ _ _ w95 _ _ _ _]
          frame "Init" {
            w40 = FALSE  # Force end
            w41 = FALSE  # Placeholder
            # "First case that is executed, executes regardless of loop beeing enabled.\nOnly executes once. Init loop data and other variables."
            n100 = Bundle("Placeholder"=w41) -> (w42:cluster{"Placeholder":bool})  [unwired: 1 in]
          }
          frame "Standby", Default {
            # "Case that is executed when the loop is not enabled. Should not be edited."
            n101 = call "emi_Wait MS with err.vi"("milliseconds to wait(0)"=u32 200, "error in (no error)"=w45) -> ("error out"=w44:errorcluster)  [unwired: 13 in]
          }
          frame "Start" {
            # "Start or restart the loop. Should perform any init code. \nOpen channel and so on. Will perform each time the system is restarted."
            n102 = call "emi_Get Debug Disp status.vi"("error in (no error)"=w50) -> ("Debug Disp"=w48:bool, "error out"=w49:errorcluster)  [unwired: 13 in]
            n103 = Not(x=w48) -> (.not. x?=w47:bool)
          }
          frame "Normal Operation" {
            # "Normal Throughput"
            n104 = call "emi_SMLoop Overview.vi"("Loop index data type"=w95, "error in (no error)"=w99) -> ("Loops"=→"Loops":T11[], "error out"=w82:errorcluster)  [unwired: 12 in]
            n105 = call "LEIN m SIC Command N.vi"("error in (no error)"=w99) -> ("queue out"=w58:refnum<queue>, "error out"=w59:errorcluster)  [unwired: 13 in]
            n106 = Get Queue Status(queue=w58, error in (no error)=w59) -> (error out=w56:errorcluster, # elements in queue=→"Til Tool cmd Q":i32)  [unwired: 1 in, 6 out]
            n107 = call "PCP SIC Command Q.vi"("error in (no error)"=w82) -> ("PCP cmd Q"=w89:refnum<queue>, "error out"=w90:errorcluster)  [unwired: 13 in]
            n108 = Get Queue Status(queue=w89, error in (no error)=w90) -> (error out=w87:errorcluster, # elements in queue=→"PCP CMD Q. Element":i32)  [unwired: 1 in, 6 out]
            n109 = call "LEIN m SIC Reply Q.vi"("error in (no error)"=w56) -> ("reply Q"=w53:refnum<queue>, "error out"=w55:errorcluster)  [unwired: 13 in]
            n110 = call "PCP SIC Command Answer Q.vi"("error in (no error)"=w87) -> ("PCP Ans Q"=w81:refnum<queue>, "PCP Ans Not"=w85:refnum<notifier>, "error out"=w91:errorcluster)  [unwired: 12 in]
            n111 = Get Queue Status(queue=w53, error in (no error)=w55) -> (# elements in queue=→"Tool reply Q":i32)  [unwired: 1 in, 7 out]
            n112 = Get Queue Status(queue=w81, error in (no error)=w91) -> (error out=w86:errorcluster, # elements in queue=→"PCP Ans Q. Element":i32)  [unwired: 1 in, 6 out]
            n113 = Get Notifier Status(notifier=w85, error in (no error)=w86) -> (current notification=→"latest notification":T2, error out=w83:errorcluster)  [unwired: 3 out]
            n114 = call "emi_Wait MS with err.vi"("milliseconds to wait(0)"=u32 250, "error in (no error)"=w83) -> ("error out"=w80:errorcluster)  [unwired: 13 in]
            n115 = call "S&E Monitor.vi"("Action(GET 250)"="Action(GET)", "Type"="Type", "error in (no error)"=w80) -> ("S&E"=w77:T8[], "error out"=w67:errorcluster)  [unwired: 11 in]
            "S&E" <- w77
            n116 = call "analog Handler.vi"("Action"=Action_Analog_Handler."GET All Values", "error in (no error)"=w67) -> ("Values"=w64:dbl[], "error out"=w66:errorcluster)  [unwired: 8 in, 4 out]
            n117 = Array Size(array=w77) -> (size(s)=→"size(s)":i32)
            n118 = call "S&E Monitor.vi"("Action(GET 250)"=Actino_S&E_monitor."Get  Alarm state", "error in (no error)"=w66) -> ("S&E"=w74:T8[], "error out"=w73:errorcluster)  [unwired: 12 in]
            n119 = for {
              tunnel: w73 -> [w110]
              tunnel: w64 -> [w109]
              tunnel: w74 -> [w107] mode=indexing
              tunnel: [w106] -> w72
              tunnel: [w105] -> w63 mode=indexing
              n120 = call "S&E Message Output.vi"("All analog ch data"=w109, "Type(File Hist)"=String_outpyt_type."Displ Stat one type", "E&S Message"=w107, "error in (no error)"=w110) -> ("String(File)"=w105:string, "error out"=w106:errorcluster)  [unwired: 9 in, 1 out]
            }
            "Alarma" <- w63
            n121 = call "S&E Monitor.vi"("Action(GET 250)"=Actino_S&E_monitor."Get Error state", "error in (no error)"=w72) -> ("S&E"=w69:T8[], "error out"=w70:errorcluster)  [unwired: 12 in]
            n122 = for {
              tunnel: w70 -> [w104]
              tunnel: w69 -> [w102] mode=indexing
              tunnel: [w101] -> w62
              tunnel: [w100] -> w68 mode=indexing
              n123 = call "S&E Message Output.vi"("Type(File Hist)"=String_outpyt_type."Displ Stat one type", "E&S Message"=w102, "error in (no error)"=w104) -> ("String(File)"=w100:string, "error out"=w101:errorcluster)  [unwired: 10 in, 1 out]
            }
            "Errors" <- w68
            n124 = call "PCP Last data GFV.vi"("error in (no error)"=w62) -> ("ms since last data"=→"ms since last data":u32, "PCP Data out"=→"PCP Data out":T4, "error out"=→"error out":errorcluster)  [unwired: 12 in]
          }
          frame "Stop" {
            # "To alow VI to exit befor \nAplicatin End.\nFor use in dialogs"
            # "Stop the loop. May be restarted later. Close interfaces and the like"
          }
          frame "Error Handling" {
            # "Loop automaticaly returns here after error is found. If error is cleared, \nLoop wil continue as normal(if was operative when error."
          }
          frame "End" {
            # "Only executes at application end has. Should performa any action the loop \nneeds to finnish. Executes only once."
          }
          frame "Post" {
            # "Only exists to pas true to loop conditional without extra VI. DO Not edit"
          }
        }
      }
      n125 = Merge Errors(w24, w23) -> (w22:errorcluster)
    }
  }
  n126 = call "emi_Dialog End.vi"("error in"=w8) -> ("error out"=w4:errorcluster)  [unwired: 14 in]
  n127 = call <vilib>:"Clear Errors.vi"("error in (no error)"=w4) -> ()  [unwired: 6 in, 1 out]
